vi "ExTestAdvDispCanvas.vi"() -> ()   [LabVIEW 2010]
uses:
  <vilib>/Platform/NI_3dgraph.lvlib
panel:
  in  "Full File Name":path
  out "error out":errorcluster
  in  "error in (no error)":errorcluster
  in  "SITKFULLDISPLAYLib.SITKFullDisplay":refnum<k7>(container)
  # "Browse match pattern is set to *.tif.  Modify this if different file type is needed."
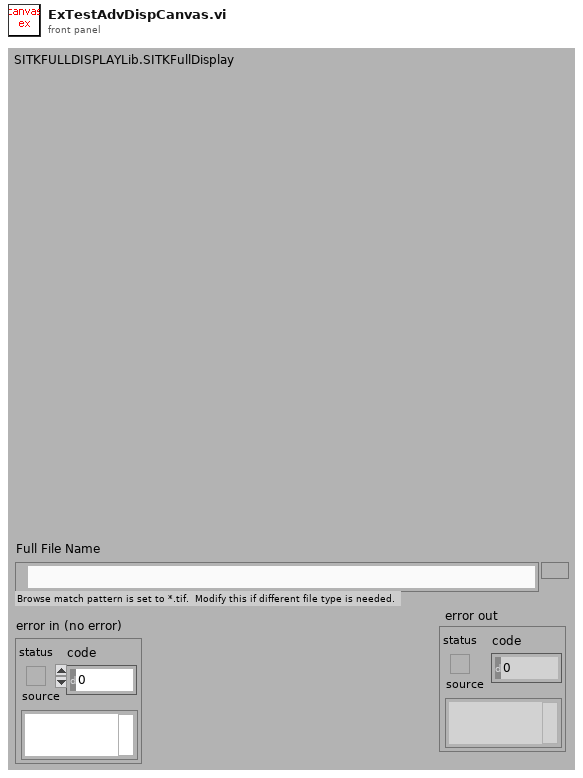
[diagram p1: front panel]
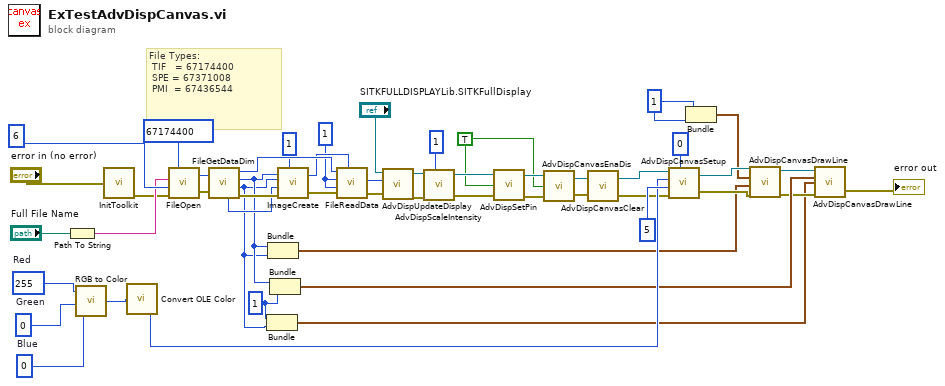
[diagram p0: block diagram]
diagram:
  w11 = 1
  w16 = 1
  w24 = 0  # Blue
  w22 = 0  # Green
  w23 = 255  # Red
  w29 = 1
  w5 = TRUE
  # "File Types:\n TIF   = 67174400\n SPE = 67371008\n PMI  = 67436544"
  n1 = Path To String(path="Full File Name") -> (string=w47:string)
  n2 = call <vilib>:"RGB to Color.vi"("B"=w24, "G"=w22, "R"=w23) -> ("Color"=w21:u32)
  n3 = call <userlib>:"InitToolkit.vi"("error in"="error in (no error)") -> ("error out"=w40:errorcluster)
  n4 = call <vilib>:"Convert OLE Color.vi"("color in"=w21) -> ("color out"=w20:u32)
  n5 = call <userlib>:"FileOpen.vi"("error in"=w40, "File Operations"=6, "FileName"=w47, "File Type"=67174400) -> ("error out"=w46:errorcluster, "File Handle"=w28:u32)
  n6 = call <userlib>:"FileGetDataDim.vi"("File Handle"=w28, "error in"=w46) -> ("Data Type"=w39:u32, "File Handle"=w44:u32, "X dim"=w13:u32, "Y dim"=w12:u32, "error out"=w45:errorcluster)  [unwired: 1 out]
  n7 = Bundle(w11, "Y dim"=w12) -> (w7:cluster{i32, "Y dim":u32})  [unwired: 1 in]
  n8 = Bundle("X dim"=w13, "Y dim"=w12) -> (w17:cluster{"X dim":u32, "Y dim":u32})  [unwired: 1 in]
  n9 = Bundle("X dim"=w13, w11) -> (w10:cluster{"X dim":u32, i32})  [unwired: 1 in]
  n10 = call <userlib>:"ImageCreate.vi"("X dimension"=w13, "Y dimension"=w12, "Data Type"=w39, "error in"=w45, "Number Of Frames"=1) -> ("Image Handle"=w42:u32, "error out"=w43:errorcluster)
  n11 = call <userlib>:"FileReadData.vi"("File Handle"=w44, "Start Frame"=w29, "End Frame"=w29, "error in"=w43, "Image Handle"=w42) -> ("Image Handle"=w32:u32, "error out"=w38:errorcluster)  [unwired: 1 out]
  n12 = call <userlib>:"AdvDispUpdateDisplay.vi"("error in (no error)"=w38, "Image Handle"=w32, "SITKFULLDISPLAYLib.SITKFullDisplay"="SITKFULLDISPLAYLib.SITKFullDisplay") -> ("error out"=w35:errorcluster, "SITKFULLDISPLAYLib.SITKFullDisplay"=w37:refnum<k7>)  [unwired: 1 in]
  n13 = call <userlib>:"AdvDispScaleIntensity.vi"("SITKFULLDISPLAYLib.SITKFullDisplay"=w37, "error in (no error)"=w35, "Type of Scale"=1) -> ("SITKFULLDISPLAYLib.SITKFullDisplay"=w36:refnum<k7>, "error out"=w34:errorcluster)  [unwired: 2 in]
  n14 = call <userlib>:"AdvDispSetPin.vi"("SITKFULLDISPLAYLib.SITKFullDisplay"=w36, "Pin Enable"=w5, "error in (no error)"=w34) -> ("SITKFULLDISPLAYLib.SITKFullDisplay"=w26:refnum<k7>, "error out"=w27:errorcluster)  [unwired: 2 out]
  n15 = call <userlib>:"AdvDispCanvasEnaDis.vi"("error in (no error)"=w27, "Canvas enable"=w5, "SITKFULLDISPLAYLib.SITKFullDisplay"=w26) -> ("error out"=w4:errorcluster, "SITKFULLDISPLAYLib.SITKFullDisplay"=w3:refnum<k7>)
  n16 = call <userlib>:"AdvDispCanvasClear.vi"("error in (no error)"=w4, "SITKFULLDISPLAYLib.SITKFullDisplay"=w3) -> ("error out"=w1:errorcluster, "SITKFULLDISPLAYLib.SITKFullDisplay"=w2:refnum<k7>)
  n17 = call <userlib>:"AdvDispCanvasSetup.vi"("SITKFULLDISPLAYLib.SITKFullDisplay"=w2, "Line Color"=w20, "Line Width"=5, "error in (no error)"=w1, "Coordinate System"=0) -> ("SITKFULLDISPLAYLib.SITKFullDisplay"=w18:refnum<k7>, "error out"=w19:errorcluster)
  n18 = Bundle(w16, w16) -> (w15:cluster{i32, i32})  [unwired: 1 in]
  n19 = call <userlib>:"AdvDispCanvasDrawLine.vi"("error in (no error)"=w19, "Point 2"=w17, "Point 1"=w15, "SITKFULLDISPLAYLib.SITKFullDisplay"=w18) -> ("error out"=w9:errorcluster, "SITKFULLDISPLAYLib.SITKFullDisplay"=w8:refnum<k7>)
  n20 = call <userlib>:"AdvDispCanvasDrawLine.vi"("error in (no error)"=w9, "Point 2"=w7, "Point 1"=w10, "SITKFULLDISPLAYLib.SITKFullDisplay"=w8) -> ("error out"=→"error out":errorcluster)  [unwired: 1 out]
